vi "Finalize To Settings.vi"(8 "error in (no error)":errorcluster, 11 "RDMA Plugin Configuration in":refnum<class "RDMA Plugin Configuration.lvclass">) -> (0 "error out":errorcluster, 2 "settings":cluster{"key":string, "value":string}[](array[cluster]), 3 "RDMA Plugin Configuration out":refnum<class "RDMA Plugin Configuration.lvclass">)   [LabVIEW 2020, in "RDMA.lvlib" / "RDMA Plugin Configuration.lvclass"]
uses:
  RDMA Plugin Configuration.lvclass
  RDMA Plugin Configuration.lvclass/RDMA Plugin Configuration.ctl
  DSF Core.lvlibp/Classes/Configuration/Configuration.lvclass
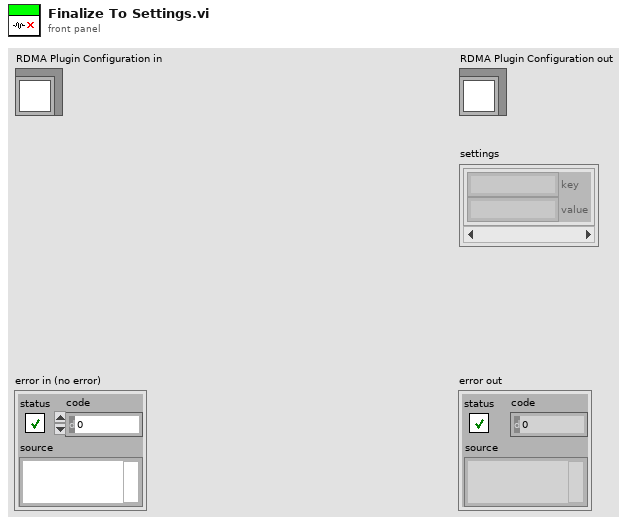
[diagram p1: front panel]
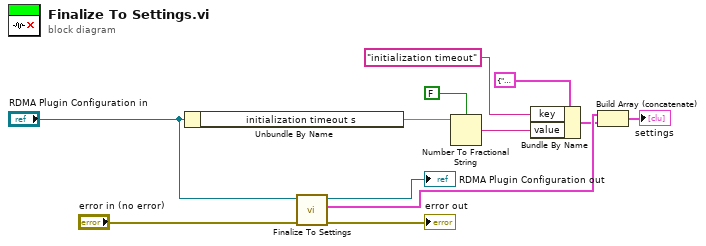
[diagram p0: block diagram]
diagram:
  n1 = Unbundle By Name("RDMA Plugin Configuration in") -> ("initialization timeout s"=w8:dbl)
  n2 = call-parent "Finalize To Settings.vi"("error in (no error)"="error in (no error)", "Configuration in"="RDMA Plugin Configuration in") -> ("error out"=→"error out":errorcluster, "settings"=w6:cluster{"key":string, "value":string}[], "Configuration out"=→"RDMA Plugin Configuration out":refnum<class "RDMA Plugin Configuration.lvclass">)  [unwired: 7 in]
  n3 = Number To Fractional String(use system decimal point (T)=FALSE, number=w8) -> (F-format string=w3:string)  [unwired: 2 in]
  n4 = Bundle By Name(cluster=cluster{"key":string, "value":string} {"key"="", "value"=""} ("setting"), "key"="initialization timeout", "value"=w3) -> (w1:cluster{"key":string, "value":string})
  n5 = Build Array (concatenate)(w6, w1) -> (→"settings":cluster{"key":string, "value":string}[])
